vi "FileIO_GetMostRecentPath.vi"(0 "Path In":path, 5 "File or Folder ?":enum16{"Folder", "File"}(ring)=enum."File", 11 "Error In":errorcluster) -> (4 "Path Out":path, 6 "Found ?":bool, 8 "Report Text":string, 15 "Error Out":errorcluster)   [LabVIEW 2016]
doc: "This VI will search and return the file/folder path for the most recent (newest) file/folder from within a given folder. If folder is empty returns empty path.\n\nAlso returns a boolean for whether or not most recent file/folder is found, along with report text if folder was empty."
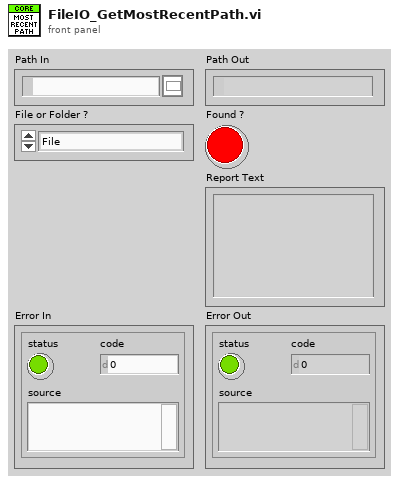
[diagram p1: front panel]
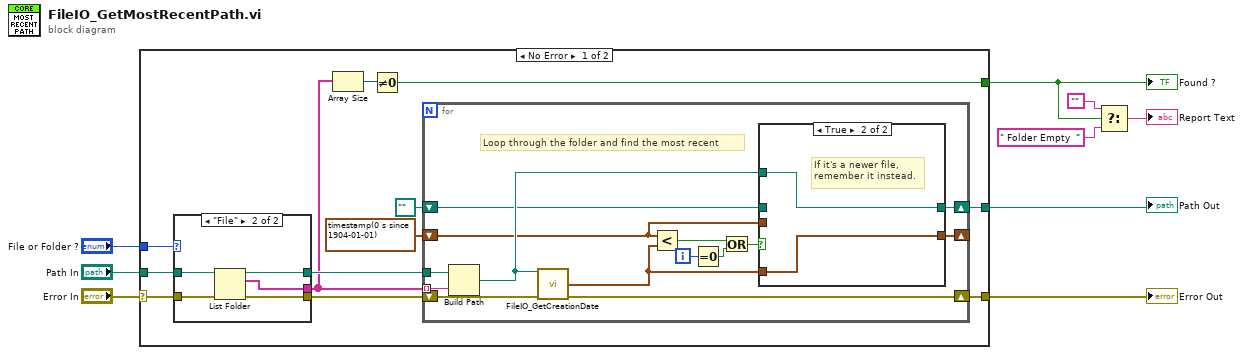
[diagram p0: block diagram]
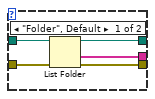
[diagram p2: hidden frame]
diagram:
  n1 = case shown="No Error" "Error In" {
    selector: "Error In" -> [w17 w50]
    tunnel: [w21 w50] -> w6
    tunnel: "Path In" -> [w15 _]
    tunnel: [w18 _] -> w5
    tunnel: "File or Folder ?" -> [w14 _]
    tunnel: [w10 _] -> w4
    frame No Error {
      n2 = case shown="\"File\"" w14 {
        tunnel: [w22 w27] -> w12
        tunnel: [w25 w31] -> w13
        tunnel: w15 -> [w26 w30]
        tunnel: w17 -> [w24 w29]
        tunnel: [w23 w28] -> w16
        frame "Folder", Default {
          n3 = List Folder(path=w26, error in=w24) -> (path out=w25:path, folder names=w22:string[], error out=w23:errorcluster)  [unwired: 2 in, 1 out]
        }
        frame "File" {
          n4 = List Folder(path=w30, error in=w29) -> (path out=w31:path, filenames=w27:string[], error out=w28:errorcluster)  [unwired: 2 in, 1 out]
        }
      }
      n5 = Array Size(array=w12) -> (size(s)=w11:i32)
      n6 = Not Equal To 0?(x=w11) -> (x != 0?=w10:bool)
      n7 = for {
        shift-right: [w40] -> _
        shift-left: timestamp(0 s since 1904-01-01) ("last mod 2") -> [w32]
        shift-right: [w38] -> w18
        shift-left: path "" -> [w37]
        shift-right: [w36] -> w21
        shift-left: w16 -> [w45]
        tunnel: w13 -> [w35]
        tunnel: w12 -> [w34] mode=indexing
        i -> [w41]
        # "Loop through the folder and find the most recent"
        n8 = Build Path(base path=w35, name or relative path=w34) -> (appended path=w39:path)
        n9 = call "FileIO_GetCreationDate.vi"("File Path"=w39, "Error In"=w45) -> ("Time Stamp Control"=w33:timestamp, "Error Out"=w36:errorcluster)  [unwired: 10 in, 2 out]
        n10 = Less?(x=w32, y=w33) -> (x < y?=w43:bool)
        n11 = Equal To 0?(x=w41) -> (x = 0?=w42:bool)
        n12 = Or(x=w43, y=w42) -> (x .or. y?=w44:bool)
        n13 = case shown="True" w44 {
          tunnel: w32 -> [w47 _]
          tunnel: [w47 w49] -> w40
          tunnel: w33 -> [_ w49]
          tunnel: w39 -> [_ w48]
          tunnel: [w46 w48] -> w38
          tunnel: w37 -> [w46 _]
          frame False {
          }
          frame True {
            # "If it's a newer file,\nremember it instead."
          }
        }
      }
    }
    frame Error {
    }
  }
  "Found ?" <- w4
  "Path Out" <- w5
  "Error Out" <- w6
  n14 = Select(t="", s=w4, f=" Folder Empty  ") -> (s? t:f=→"Report Text":string)
